vi "filter_vial_No.vi"() -> ()   [LabVIEW 2020]
panel:
  in  "filter_vial_No":i32
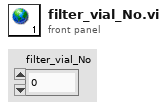
[diagram p1: front panel]
diagram:
